vi "ReadDirection.vi"(0 "object in":refnum<class "Game Board.lvclass">, 2 "Direction SEQ":refnum<queue>, 5 "error in (no error)":errorcluster) -> (14 "object out":refnum<class "Game Board.lvclass">, 19 "error out":errorcluster)   [LabVIEW 2021, in "Game Board.lvclass"]
uses:
  Game Board.lvclass
  Direction.ctl
  Game Board.lvclass/Game Board.ctl
  Snake_class/Snake.lvclass
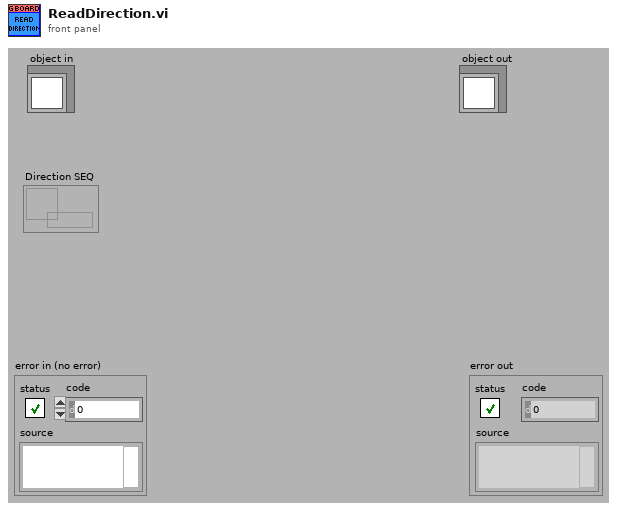
[diagram p1: front panel]
types:
  T1 = typedef "Direction.ctl" = enum16{"up", "down", "left", "right"}
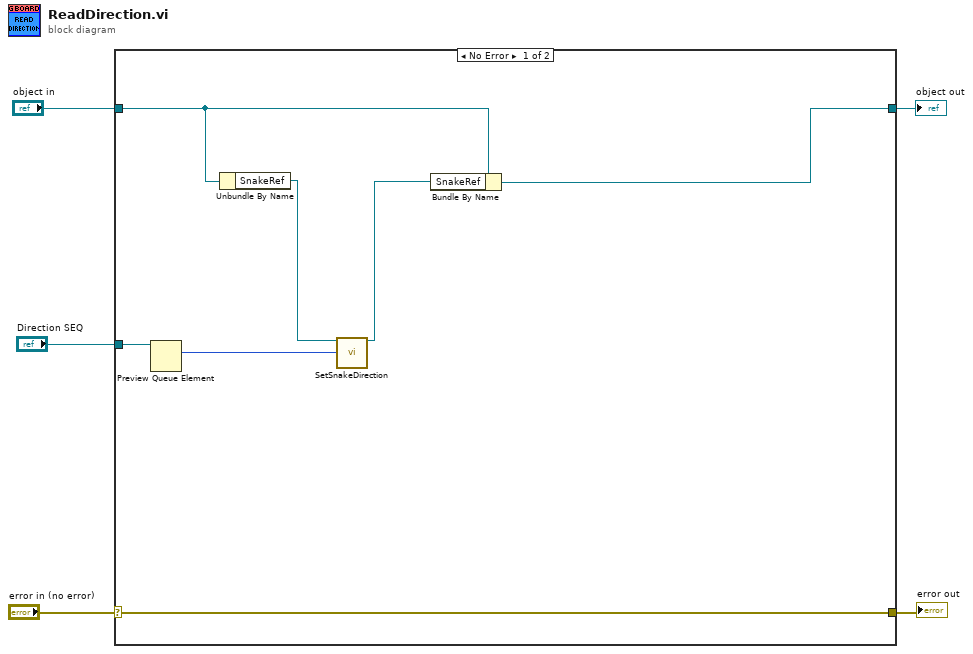
[diagram p0: block diagram]
diagram:
  n1 = case shown="No Error" "error in (no error)" {
    selector: "error in (no error)" -> [w12 w14]
    tunnel: [w12 w14] -> w4
    tunnel: [w7 w13] -> w2
    tunnel: "object in" -> [w8 w13]
    tunnel: "Direction SEQ" -> [w11 _]
    frame No Error {
      n2 = Preview Queue Element(queue=w11) -> (element=w6:T1)  [unwired: 2 in, 3 out]
      n3 = Unbundle By Name(w8) -> ("SnakeRef"=w10:refnum<class "Snake.lvclass">)
      n4 = call-dynamic "SetSnakeDirection.vi"("object in"=w10, "Direction"=w6) -> ("object out"=w9:refnum<class "Snake.lvclass">)  [unwired: 16 in, 1 out]
      n5 = Bundle By Name(cluster=w8, "SnakeRef"=w9) -> (w7:refnum<class "Game Board.lvclass">)
    }
    frame Error {
    }
  }
  "error out" <- w4
  "object out" <- w2
